vi "Value Change.vi"(8 "error in (no error)":errorcluster, 9 "New":T1, 10 "Old":T1, 11 "BluelinesRedlines in":refnum<class "BluelinesRedlines.lvclass">) -> (0 "error out":errorcluster, 3 "BluelinesRedlines out":refnum<class "BluelinesRedlines.lvclass">)   [LabVIEW 2020, in "VolatusGUIElements.lvlib" / "BluelinesRedlines.lvclass"]
uses:
  BluelinesRedlines.lvclass
  BluelinesRedlines.lvclass/BluelinesRedlines.ctl
  VolatusGUI/BluelinesRedlines Source/BLRL Type.ctl
  VolatusGUI/BluelinesRedlines Source/BluelinesRedlines Source.lvclass
  Volatus/VolatusAPI/VolatusAPI.lvclass
  BLRL Control.ctl
panel:
  # "Low"
  # "Value"
  # "High"
  # "Low"
  # "Value"
  # "High"
  # "Low"
  # "Value"
  # "High"
  # "Low"
  # "Value"
  # "High"
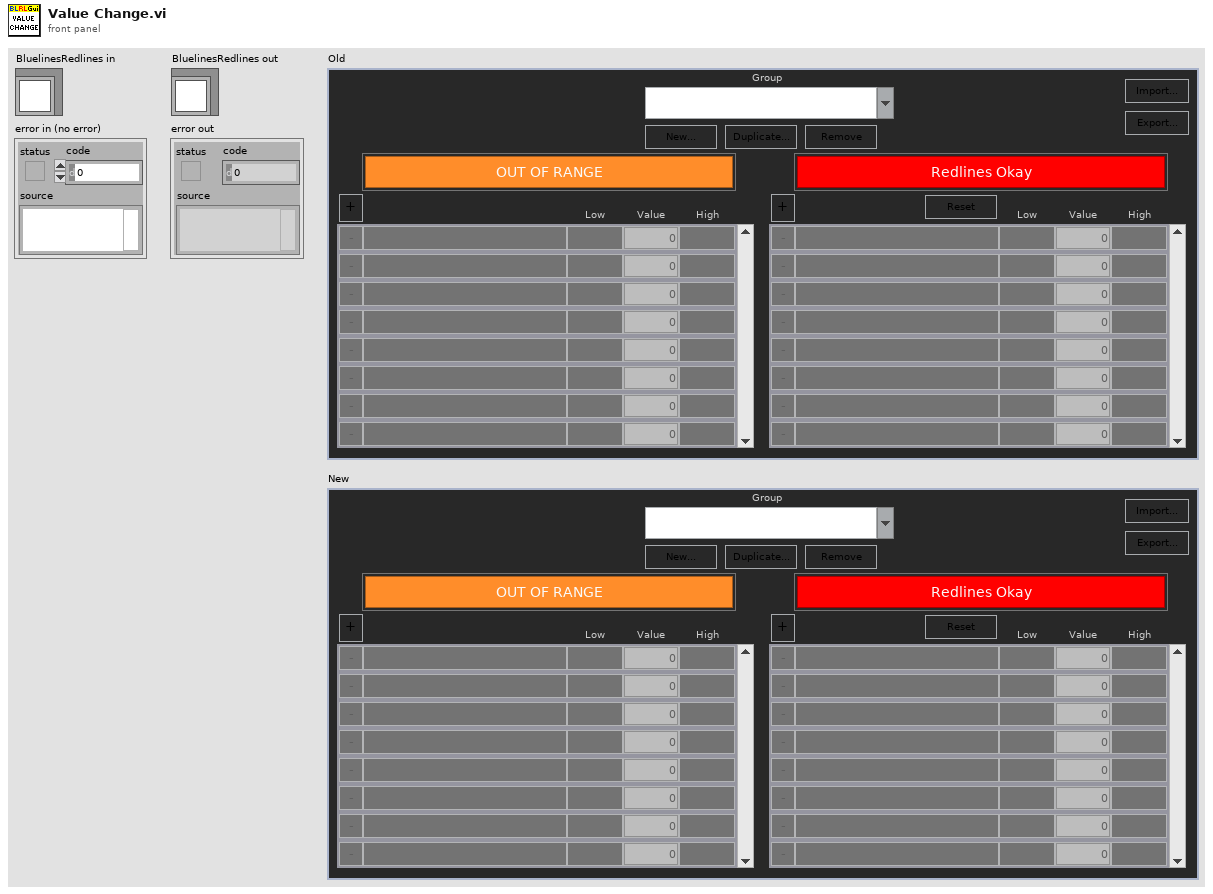
[diagram p1: front panel]
types:
  T1 = typedef "VolatusGUIElements.lvlib/BluelinesRedlines.lvclass/BLRL Control.ctl" = cluster{"Blue Lines":cluster{"Channel":string, "Low":string, "Value":dbl, "High":string, "Color":u32, "Remove Channel":bool}[], "Red Lines":cluster{"Channel":string, "Low":string, "Value":dbl, "High":string, "Color":u32, "Remove Channel":bool}[], "Import":bool, "Export":bool, "Blueline Status":bool, "Redlines Status":bool, "Group":string, "New Group":bool, "Dup Group":bool, "Remove Group":bool, "Add Blue Channel":bool, "Add Red Channel":bool, "Reset Redlines":bool}
  T2 = cluster{"Blue Lines":cluster{"Channel":bool, "Low":bool, "Value":bool, "High":bool, "Color":bool, "Remove Channel":bool}[], "Red Lines":cluster{"Channel":bool, "Low":bool, "Value":bool, "High":bool, "Color":bool, "Remove Channel":bool}[], "Import":bool, "Export":bool, "Blueline Status":bool, "Redlines Status":bool, "Group":bool, "New Group":bool, "Dup Group":bool, "Remove Group":bool, "Add Blue Channel":bool, "Add Red Channel":bool, "Reset Redlines":bool}
  T3 = typedef "VolatusGUI.lvlib/BluelinesRedlines Source.lvclass/BLRL Type.ctl" = enum16{"Blueline", "Redline"}
  T4 = cluster{"Channel":string, "Low":string, "Value":dbl, "High":string, "Color":u32, "Remove Channel":bool}[]
  T5 = cluster{"Channel":bool, "Low":bool, "Value":bool, "High":bool, "Color":bool, "Remove Channel":bool}[]
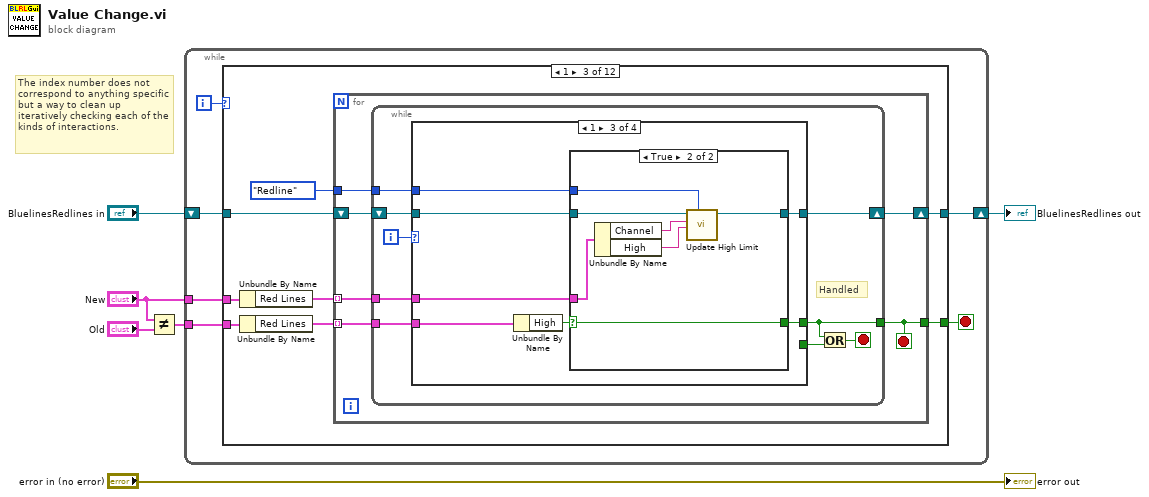
[diagram p0: block diagram]
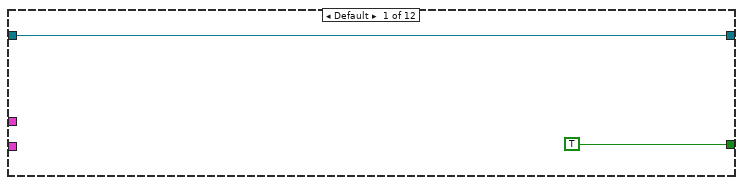
[diagram p2: hidden frame]
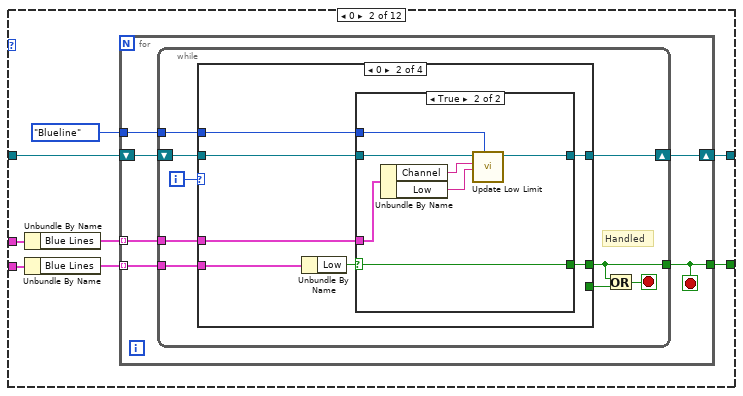
[diagram p3: hidden frame]
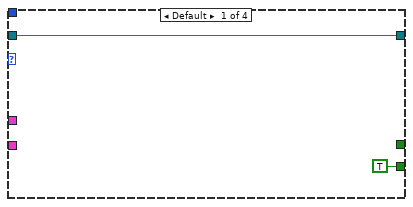
[diagram p4: hidden frame]
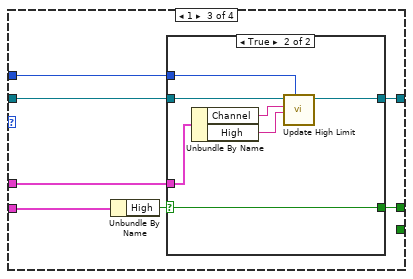
[diagram p6: hidden frame]
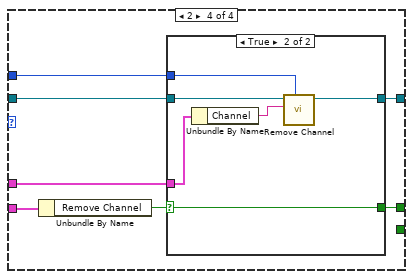
[diagram p8: hidden frame]
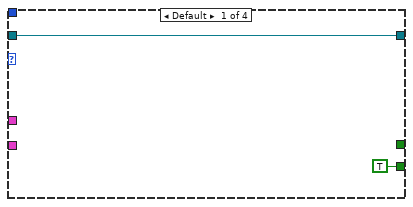
[diagram p10: hidden frame]
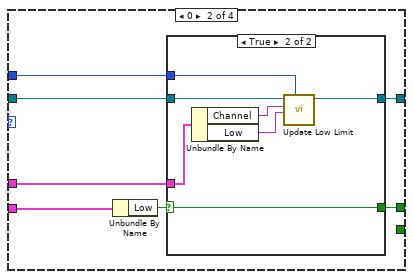
[diagram p11: hidden frame]
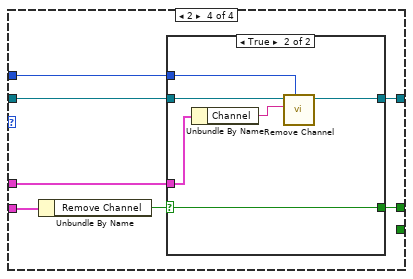
[diagram p14: hidden frame]
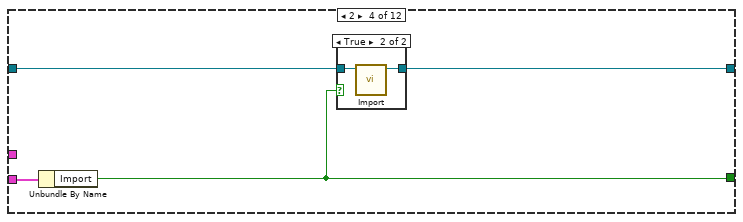
[diagram p16: hidden frame]
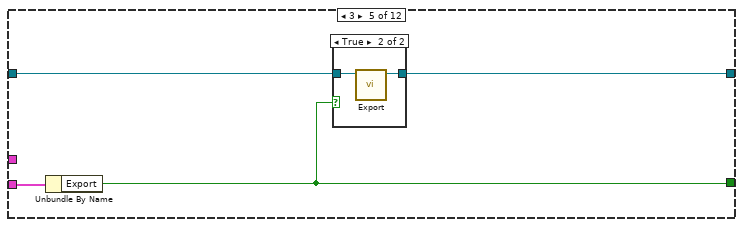
[diagram p18: hidden frame]
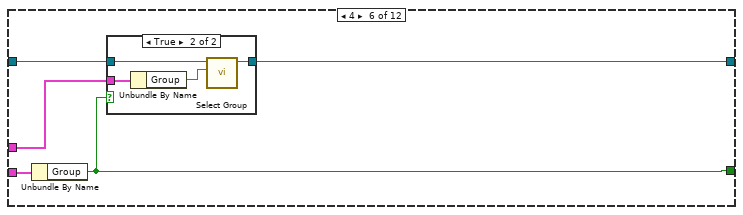
[diagram p20: hidden frame]
diagram:
  # "The index number does not correspond to anything specific but a way to clean up iteratively checking each of the kinds of interactions."
  n1 = Not Equal?(x="New", y="Old") -> (x != y?=w4:T2)
  n2 = while {
    tunnel: w4 -> [w8]
    shift-right: [w11] -> w2
    shift-left: "BluelinesRedlines in" -> [w10]
    tunnel: "New" -> [w7]
    i -> [w12]
    stop <- w9 stop-if-true
    n3 = case shown="1" w12 {
      tunnel: [w14 w17 w86 w154 w161 w168 w178 w188 w195 w202 w210 w218] -> w11
      tunnel: w10 -> [w14 w20 w89 w156 w163 w170 w179 w190 w197 w204 w212 w220]
      tunnel: [TRUE w16 w85 w153 w160 w167 w177 w187 w194 w201 w209 w217] -> w9
      tunnel: w8 -> [_ w22 w91 w155 w162 w171 w180 w189 w196 w203 w211 w219]
      tunnel: w7 -> [_ w19 w88 _ _ w169 _ _ _ _ _ _]
      frame Default {
      }
      frame 0 {
        n4 = Unbundle By Name(w19) -> ("Blue Lines"=w18:T4)
        n5 = Unbundle By Name(w22) -> ("Blue Lines"=w21:T5)
        n6 = for {
          tunnel: w21 -> [w26] mode=indexing
          shift-right: [w27] -> w17
          shift-left: w20 -> [w28]
          tunnel: w18 -> [w25] mode=indexing
          tunnel: [w24] -> w16
          tunnel: BLRL_Type."Blueline" ("BLRL Type") -> [w23]
          stop <- w24 stop-if-true
          n7 = while {
            shift-right: [w37] -> w27
            shift-left: w28 -> [w36]
            tunnel: w26 -> [w34]
            tunnel: w25 -> [w33]
            tunnel: [w31] -> w24
            tunnel: w23 -> [w29]
            i -> [w35]
            stop <- w32 stop-if-true
            # "Handled"
            n8 = case shown="0" w35 {
              tunnel: [w38 w42 w57 w72] -> w37
              tunnel: w36 -> [w38 w41 w56 w71]
              tunnel: w34 -> [_ w46 w61 w76]
              tunnel: w33 -> [_ w44 w59 w74]
              tunnel: [_ w43 w58 w73] -> w31
              tunnel: [TRUE _ _ _] -> w30
              tunnel: w29 -> [_ w40 w55 w70]
              frame Default {
              }
              frame 0 {
                n9 = Unbundle By Name(w46) -> ("Low"=w45:bool)
                n10 = case shown="True" w45 {
                  selector: w45 -> [_ w54]
                  tunnel: w44 -> [_ w52]
                  tunnel: [_ w54] -> w43
                  tunnel: [w47 w51] -> w42
                  tunnel: w41 -> [w47 w53]
                  tunnel: w40 -> [_ w48]
                  frame False {
                  }
                  frame True {
                    n11 = Unbundle By Name(w52) -> ("Channel"=w50:string, "Low"=w49:string)
                    n12 = call "Update Low Limit.vi"("BLRL Type"=w48, "Low Limit"=w49, "Channel"=w50, "BluelinesRedlines in"=w53) -> ("BluelinesRedlines out"=w51:refnum<class "BluelinesRedlines.lvclass">)  [unwired: 6 in, 1 out]
                  }
                }
              }
              frame 1 {
                n13 = Unbundle By Name(w61) -> ("High"=w60:bool)
                n14 = case shown="False" w60 {
                  selector: w60 -> [_ w69]
                  tunnel: w59 -> [_ w67]
                  tunnel: [_ w69] -> w58
                  tunnel: [w62 w66] -> w57
                  tunnel: w56 -> [w62 w68]
                  tunnel: w55 -> [_ w63]
                  frame False {
                  }
                  frame True {
                    n15 = Unbundle By Name(w67) -> ("Channel"=w65:string, "High"=w64:string)
                    n16 = call "Update High Limit.vi"("BLRL Type"=w63, "High Limit"=w64, "Channel"=w65, "BluelinesRedlines in"=w68) -> ("BluelinesRedlines out"=w66:refnum<class "BluelinesRedlines.lvclass">)  [unwired: 6 in, 1 out]
                  }
                }
              }
              frame 2 {
                n17 = Unbundle By Name(w76) -> ("Remove Channel"=w75:bool)
                n18 = case shown="False" w75 {
                  selector: w75 -> [_ w83]
                  tunnel: w74 -> [_ w81]
                  tunnel: [_ w83] -> w73
                  tunnel: [w77 w80] -> w72
                  tunnel: w71 -> [w77 w82]
                  tunnel: w70 -> [_ w78]
                  frame False {
                  }
                  frame True {
                    n19 = Unbundle By Name(w81) -> ("Channel"=w79:string)
                    n20 = call "Remove Channel.vi"("BLRL Type"=w78, "Channel"=w79, "BluelinesRedlines in"=w82) -> ("BluelinesRedlines out"=w80:refnum<class "BluelinesRedlines.lvclass">)  [unwired: 7 in, 1 out]
                  }
                }
              }
            }
            n21 = Or(x=w31, y=w30) -> (x .or. y?=w32:bool)
          }
        }
      }
      frame 1 {
        n22 = Unbundle By Name(w88) -> ("Red Lines"=w87:T4)
        n23 = Unbundle By Name(w91) -> ("Red Lines"=w90:T5)
        n24 = for {
          tunnel: w90 -> [w95] mode=indexing
          shift-right: [w96] -> w86
          shift-left: w89 -> [w97]
          tunnel: w87 -> [w94] mode=indexing
          tunnel: [w93] -> w85
          tunnel: BLRL_Type."Redline" ("BLRL Type") -> [w92]
          stop <- w93 stop-if-true
          n25 = while {
            shift-right: [w106] -> w96
            shift-left: w97 -> [w105]
            tunnel: w95 -> [w103]
            tunnel: w94 -> [w102]
            tunnel: [w100] -> w93
            tunnel: w92 -> [w98]
            i -> [w104]
            stop <- w101 stop-if-true
            # "Handled"
            n26 = case shown="1" w104 {
              tunnel: [w107 w111 w126 w141] -> w106
              tunnel: w105 -> [w107 w110 w125 w140]
              tunnel: w103 -> [_ w115 w130 w145]
              tunnel: w102 -> [_ w113 w128 w143]
              tunnel: [_ w112 w127 w142] -> w100
              tunnel: [TRUE _ _ _] -> w99
              tunnel: w98 -> [_ w109 w124 w139]
              frame Default {
              }
              frame 0 {
                n27 = Unbundle By Name(w115) -> ("Low"=w114:bool)
                n28 = case shown="True" w114 {
                  selector: w114 -> [_ w123]
                  tunnel: w113 -> [_ w121]
                  tunnel: [_ w123] -> w112
                  tunnel: [w116 w120] -> w111
                  tunnel: w110 -> [w116 w122]
                  tunnel: w109 -> [_ w117]
                  frame False {
                  }
                  frame True {
                    n29 = Unbundle By Name(w121) -> ("Channel"=w119:string, "Low"=w118:string)
                    n30 = call "Update Low Limit.vi"("BLRL Type"=w117, "Low Limit"=w118, "Channel"=w119, "BluelinesRedlines in"=w122) -> ("BluelinesRedlines out"=w120:refnum<class "BluelinesRedlines.lvclass">)  [unwired: 6 in, 1 out]
                  }
                }
              }
              frame 1 {
                n31 = Unbundle By Name(w130) -> ("High"=w129:bool)
                n32 = case shown="True" w129 {
                  selector: w129 -> [_ w138]
                  tunnel: w128 -> [_ w136]
                  tunnel: [_ w138] -> w127
                  tunnel: [w131 w135] -> w126
                  tunnel: w125 -> [w131 w137]
                  tunnel: w124 -> [_ w132]
                  frame False {
                  }
                  frame True {
                    n33 = Unbundle By Name(w136) -> ("Channel"=w134:string, "High"=w133:string)
                    n34 = call "Update High Limit.vi"("BLRL Type"=w132, "High Limit"=w133, "Channel"=w134, "BluelinesRedlines in"=w137) -> ("BluelinesRedlines out"=w135:refnum<class "BluelinesRedlines.lvclass">)  [unwired: 6 in, 1 out]
                  }
                }
              }
              frame 2 {
                n35 = Unbundle By Name(w145) -> ("Remove Channel"=w144:bool)
                n36 = case shown="True" w144 {
                  selector: w144 -> [_ w152]
                  tunnel: w143 -> [_ w150]
                  tunnel: [_ w152] -> w142
                  tunnel: [w146 w149] -> w141
                  tunnel: w140 -> [w146 w151]
                  tunnel: w139 -> [_ w147]
                  frame False {
                  }
                  frame True {
                    n37 = Unbundle By Name(w150) -> ("Channel"=w148:string)
                    n38 = call "Remove Channel.vi"("BLRL Type"=w147, "Channel"=w148, "BluelinesRedlines in"=w151) -> ("BluelinesRedlines out"=w149:refnum<class "BluelinesRedlines.lvclass">)  [unwired: 7 in, 1 out]
                  }
                }
              }
            }
            n39 = Or(x=w100, y=w99) -> (x .or. y?=w101:bool)
          }
        }
      }
      frame 2 {
        n40 = Unbundle By Name(w155) -> ("Import"=w153:bool)
        n41 = case shown="True" w153 {
          tunnel: w156 -> [w157 w159]
          tunnel: [w157 w158] -> w154
          frame False {
          }
          frame True {
            n42 = call "Import.vi"("BluelinesRedlines in"=w159) -> ("BluelinesRedlines out"=w158:refnum<class "BluelinesRedlines.lvclass">)  [unwired: 9 in, 1 out]
          }
        }
      }
      frame 3 {
        n43 = Unbundle By Name(w162) -> ("Export"=w160:bool)
        n44 = case shown="True" w160 {
          tunnel: w163 -> [w164 w166]
          tunnel: [w164 w165] -> w161
          frame False {
          }
          frame True {
            n45 = call "Export.vi"("BluelinesRedlines in"=w166) -> ("BluelinesRedlines out"=w165:refnum<class "BluelinesRedlines.lvclass">)  [unwired: 9 in, 1 out]
          }
        }
      }
      frame 4 {
        n46 = Unbundle By Name(w171) -> ("Group"=w167:bool)
        n47 = case shown="True" w167 {
          tunnel: w170 -> [w172 w175]
          tunnel: w169 -> [_ w176]
          tunnel: [w172 w173] -> w168
          frame False {
          }
          frame True {
            n48 = Unbundle By Name(w176) -> ("Group"=w174:string)
            n49 = call "Select Group.vi"("Group"=w174, "BluelinesRedlines in"=w175) -> ("BluelinesRedlines out"=w173:refnum<class "BluelinesRedlines.lvclass">)  [unwired: 8 in, 1 out]
          }
        }
      }
      frame 5 {
        n50 = Unbundle By Name(w180) -> ("New Group"=w177:bool)
        n51 = case shown="True" w177 {
          tunnel: w179 -> [w181 w185]
          tunnel: [w181 w186] -> w178
          frame False {
          }
          frame True {
            n52 = call "New Group.vi"("BluelinesRedlines in"=w185) -> ("error out"=w183:errorcluster, "BluelinesRedlines out"=w186:refnum<class "BluelinesRedlines.lvclass">)  [unwired: 9 in]
            n53 = Unbundle By Name(w185) -> ("VolatusAPI"=w184:refnum<class "VolatusAPI.lvclass">)
            n54 = call <vilib>:"Simple Error Handler.vi"("error in (no error)"=w183) -> ()  [unwired: 4 in, 5 out]
            n55 = call "Report Error.vi"("error in (no error)"=w183, "Context"="New BLRL group", "VolatusAPI in"=w184) -> ()  [unwired: 7 in, 2 out]
          }
        }
      }
      frame 6 {
        n56 = Unbundle By Name(w189) -> ("Dup Group"=w187:bool)
        n57 = case shown="True" w187 {
          tunnel: w190 -> [w191 w193]
          tunnel: [w191 w192] -> w188
          frame False {
          }
          frame True {
            n58 = call "Duplicate Group.vi"("BluelinesRedlines in"=w193) -> ("BluelinesRedlines out"=w192:refnum<class "BluelinesRedlines.lvclass">)  [unwired: 9 in, 1 out]
          }
        }
      }
      frame 7 {
        n59 = Unbundle By Name(w196) -> ("Remove Group"=w194:bool)
        n60 = case shown="True" w194 {
          tunnel: w197 -> [w198 w200]
          tunnel: [w198 w199] -> w195
          frame False {
          }
          frame True {
            n61 = call "Remove Group.vi"("BluelinesRedlines in"=w200) -> ("BluelinesRedlines out"=w199:refnum<class "BluelinesRedlines.lvclass">)  [unwired: 9 in, 1 out]
          }
        }
      }
      frame 8 {
        n62 = Unbundle By Name(w203) -> ("Add Blue Channel"=w201:bool)
        n63 = case shown="True" w201 {
          tunnel: w204 -> [w205 w208]
          tunnel: [w205 w207] -> w202
          frame False {
          }
          frame True {
            n64 = call "Add Channel.vi"("BLRL Type"=BLRL_Type."Blueline", "BluelinesRedlines in"=w208) -> ("BluelinesRedlines out"=w207:refnum<class "BluelinesRedlines.lvclass">)  [unwired: 8 in, 1 out]
          }
        }
      }
      frame 9 {
        n65 = Unbundle By Name(w211) -> ("Add Red Channel"=w209:bool)
        n66 = case shown="True" w209 {
          tunnel: w212 -> [w213 w216]
          tunnel: [w213 w215] -> w210
          frame False {
          }
          frame True {
            n67 = call "Add Channel.vi"("BLRL Type"=BLRL_Type."Redline", "BluelinesRedlines in"=w216) -> ("BluelinesRedlines out"=w215:refnum<class "BluelinesRedlines.lvclass">)  [unwired: 8 in, 1 out]
          }
        }
      }
      frame 10 {
        n68 = Unbundle By Name(w219) -> ("Reset Redlines"=w217:bool)
        n69 = case shown="True" w217 {
          tunnel: w220 -> [w221 w223]
          tunnel: [w221 w222] -> w218
          frame False {
          }
          frame True {
            n70 = call "Reset Redlines.vi"("BluelinesRedlines in"=w223) -> ("BluelinesRedlines out"=w222:refnum<class "BluelinesRedlines.lvclass">)  [unwired: 9 in, 1 out]
          }
        }
      }
    }
  }
  "BluelinesRedlines out" <- w2
  "error out" <- "error in (no error)"
